vi "Global 2.vi"() -> ()   [LabVIEW 2019]
panel:
  out "G_Sample_Set":dbl
  out "Sample_Stab":bool
  out "Remote_T_Ramp":bool
  in  "Remote_T_Rate":dbl
  in  "Remote_T_Set":dbl
  out "Remote_T_Run":bool
  out "Remote_T_GoTo":bool
  out "VTI_Temp":dbl
  out "SampleTemp":dbl
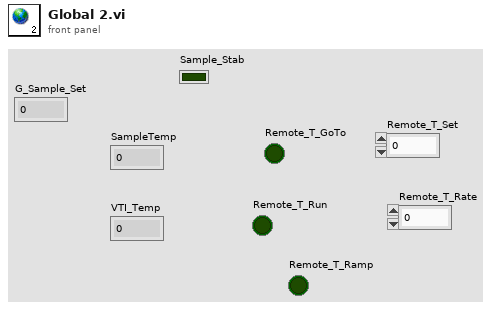
[diagram p1: front panel]
diagram:
